vi "flatten_tester.vi"() -> ()   [LabVIEW 2020]
uses:
  shared/message--cluster.ctl
  shared/request--enum.ctl
panel:
  out "value":T1
  out "data string":string
  out "error out":errorcluster
  in  "request":T1
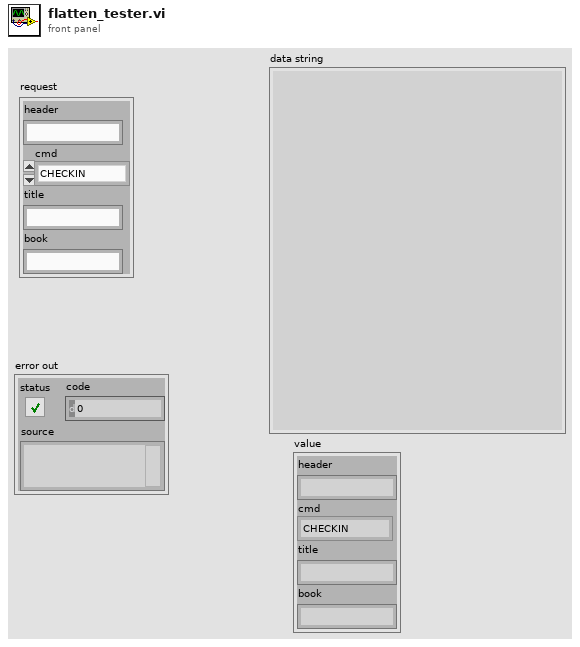
[diagram p1: front panel]
types:
  T1 = typedef "message--cluster.ctl" = cluster{"header":string, "cmd":T2, "title":string, "book":string}
  T2 = typedef "request--enum.ctl" = enum16{"CHECKIN", "CHECKOUT"}
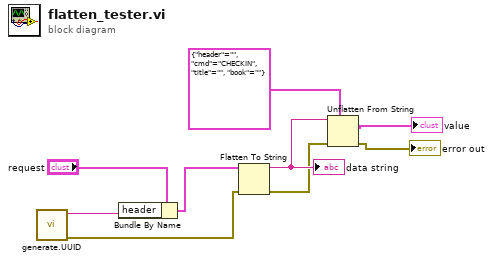
[diagram p0: block diagram]
diagram:
  n1 = call "generate.UUID.vi"() -> ("error out"=w6:errorcluster, "UUID"=w7:string)  [unwired: 10 in]
  n2 = Bundle By Name(cluster="request", "header"=w7) -> (w8:T1)
  n3 = Flatten To String(anything=w8, error in (no error)=w6) -> (data string=w5:string, error out=w2:errorcluster)  [unwired: 2 in, 1 out]
  "data string" <- w5
  n4 = Unflatten From String(type=T1 {"header"="", "cmd"=enum."CHECKIN", "title"="", "book"=""} ("request"), binary string=w5, error in (no error)=w2) -> (value=→"value":T1, error out=→"error out":errorcluster)  [unwired: 2 in, 1 out]
